vi "Write New Image.vi"(8 "error in (no error)":errorcluster, 10 "Image":T1, 11 "Camara in":refnum<class "Camara.lvclass">) -> (0 "error out":errorcluster, 3 "Camara out":refnum<class "Camara.lvclass">)   [LabVIEW 2020, in "Camara.lvclass"]
uses:
  Camara.lvclass
  <vilib>/vision/Image Controls.llb/IMAQ Image.ctl
  Camara.lvclass/Camara.ctl
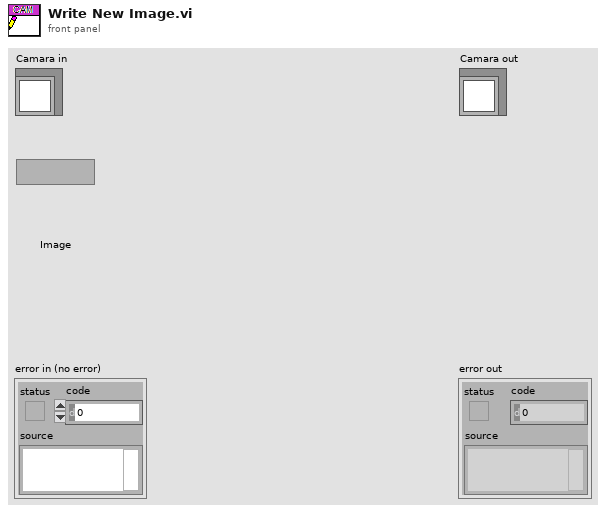
[diagram p1: front panel]
types:
  T1 = typedef "IMAQ Image.ctl" = refnum<image>
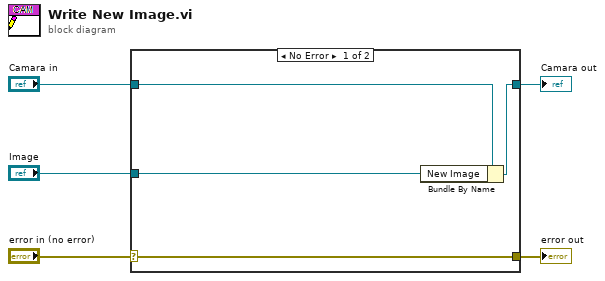
[diagram p0: block diagram]
diagram:
  n1 = case shown="No Error" "error in (no error)" {
    selector: "error in (no error)" -> [w9 w10]
    tunnel: [w9 w10] -> w4
    tunnel: [w7 w11] -> w2
    tunnel: "Camara in" -> [w8 w11]
    tunnel: "Image" -> [w6 _]
    frame No Error {
      n2 = Bundle By Name(cluster=w8, "New Image"=w6) -> (w7:refnum<class "Camara.lvclass">)
    }
    frame Error {
    }
  }
  "error out" <- w4
  "Camara out" <- w2
